vi "Coef-Temp to color convert.vi"() -> ()   [LabVIEW 2018]
uses:
  Coef-Temp-.ctl
  Resistor Band Colors.lvlib
panel:
  in  "Coef. Temp.":T1
  out "Color":u32
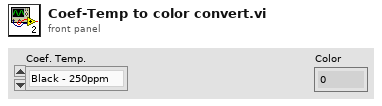
[diagram p1: front panel]
types:
  T1 = typedef "Coef-Temp-.ctl" = enum16{"Black - 250ppm", "Brown - 100ppm", "Red - 50ppm", "Orange - 15ppm", "Yellow - 25ppm", "Green - 20ppm", "Blue - 10ppm", "Violet - 5ppm"}
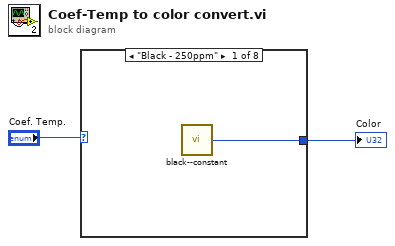
[diagram p0: block diagram]
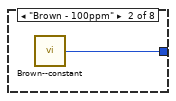
[diagram p2: hidden frame]
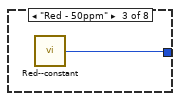
[diagram p3: hidden frame]
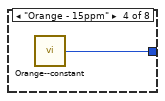
[diagram p4: hidden frame]
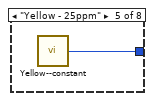
[diagram p5: hidden frame]
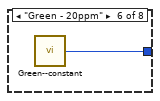
[diagram p6: hidden frame]
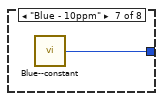
[diagram p7: hidden frame]
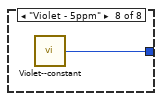
[diagram p8: hidden frame]
diagram:
  n1 = case shown="\"Black - 250ppm\"" "Coef. Temp." {
    tunnel: [w3 w4 w5 w6 w7 w8 w9 w10] -> w2
    frame "Black - 250ppm" {
      n2 = call "black--constant.vi"() -> ("Color"=w3:u32)  [unwired: 5 in]
    }
    frame "Brown - 100ppm" {
      n3 = call "Brown--constant.vi"() -> ("Color"=w4:u32)  [unwired: 5 in]
    }
    frame "Red - 50ppm" {
      n4 = call "Red--constant.vi"() -> ("Color"=w5:u32)  [unwired: 5 in]
    }
    frame "Orange - 15ppm" {
      n5 = call "Orange--constant.vi"() -> ("Color"=w6:u32)  [unwired: 5 in]
    }
    frame "Yellow - 25ppm" {
      n6 = call "Yellow--constant.vi"() -> ("Color"=w7:u32)  [unwired: 5 in]
    }
    frame "Green - 20ppm" {
      n7 = call "Green--constant.vi"() -> ("Color"=w8:u32)  [unwired: 5 in]
    }
    frame "Blue - 10ppm" {
      n8 = call "Blue--constant.vi"() -> ("Color"=w9:u32)  [unwired: 5 in]
    }
    frame "Violet - 5ppm" {
      n9 = call "Violet--constant.vi"() -> ("Color"=w10:u32)  [unwired: 5 in]
    }
  }
  "Color" <- w2
